vi "UpdateSpeed.vi"(6 "Attrs in":T1, 7 "Ctrl in":u32, 8 "error in":errorcluster, 10 "Attrs array in":T1[](array[typedef]), 11 "Ctrl array in":u32[](array[numeric])) -> (0 "error out":errorcluster, 2 "Attrs array out":T1[](array[typedef]), 3 "Ctrl array out":u32[](array[numeric]))   [LabVIEW 2012, in "Spinner.xctl"]
uses:
  Spinner.xctl
  Attrs.ctl
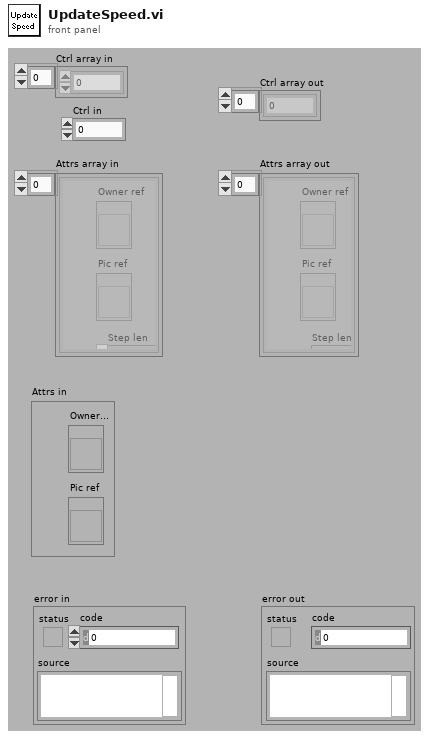
[diagram p1: front panel]
types:
  T1 = typedef "Spinner.xctl/Attrs.ctl" = cluster{"Owner ref":refnum<vi>, "Pic ref":refnum<vi>, "Step len":dbl, "Imgs":picture[], "Current phase":dbl}
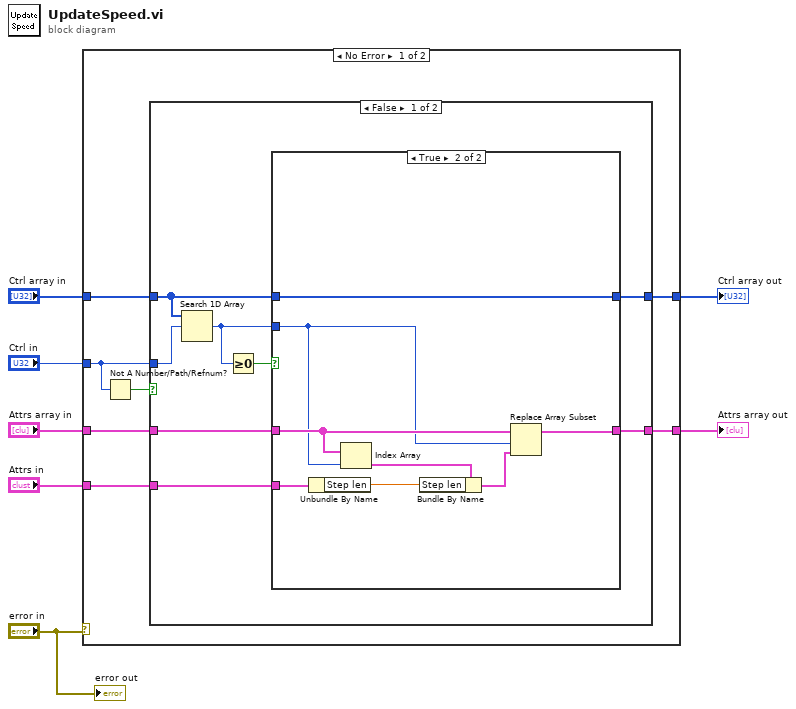
[diagram p0: block diagram]
diagram:
  n1 = case shown="No Error" "error in" {
    tunnel: "Ctrl in" -> [w12 _]
    tunnel: "Ctrl array in" -> [w13 w36]
    tunnel: "Attrs array in" -> [w11 w35]
    tunnel: "Attrs in" -> [w10 _]
    tunnel: [w9 w35] -> w3
    tunnel: [w8 w36] -> w2
    frame No Error {
      n2 = Not A Number/Path/Refnum?(number/path/refnum=w12) -> (NaN/Path/Refnum?=w14:bool)
      n3 = case shown="False" w14 {
        tunnel: w13 -> [w18 w34]
        tunnel: w12 -> [w17 _]
        tunnel: w11 -> [w21 w33]
        tunnel: w10 -> [w20 _]
        tunnel: [w19 w33] -> w9
        tunnel: [w16 w34] -> w8
        frame False {
          n4 = Search 1D Array(1D array=w18, element=w17) -> (index of element=w15:i32)  [unwired: 1 in]
          n5 = Greater Or Equal To 0?(x=w15) -> (x >= 0?=w22:bool)
          n6 = case shown="True" w22 {
            tunnel: w21 -> [w23 w28]
            tunnel: w20 -> [_ w30]
            tunnel: [w23 w27] -> w19
            tunnel: w18 -> [w24 w32]
            tunnel: [w24 w32] -> w16
            tunnel: w15 -> [_ w25]
            frame False {
            }
            frame True {
              n7 = Unbundle By Name(w30) -> ("Step len"=w29:dbl)
              n8 = Index Array(array=w28, index=w25) -> (element=w31:T1)
              n9 = Bundle By Name(cluster=w31, "Step len"=w29) -> (w26:T1)
              n10 = Replace Array Subset(array=w28, new element=w26, index=w25) -> (w27:T1[])
            }
          }
        }
        frame True {
        }
      }
    }
    frame Error {
    }
  }
  "Attrs array out" <- w3
  "Ctrl array out" <- w2
  "error out" <- "error in"
